vi "Find Non Part Signal Indexes.vi"(0 "All Type Info":T1, 5 "Channels":T3[](array[typedef])) -> (4 "Total Channel Indexes":i32[](array[numeric]), 6 "Non Part Indexes (data)":i32[](array[numeric]), 8 "Non Part Indexes (description)":i32[](array[numeric]))   [LabVIEW 2023]
uses:
  Type Defs and Controls/Channel Config.ctl
  Type Defs and Controls/All Part Info.ctl
  Type Defs and Controls/Part Info.ctl
panel:
  out "Part Channel Indexes":u16[](array[numeric])
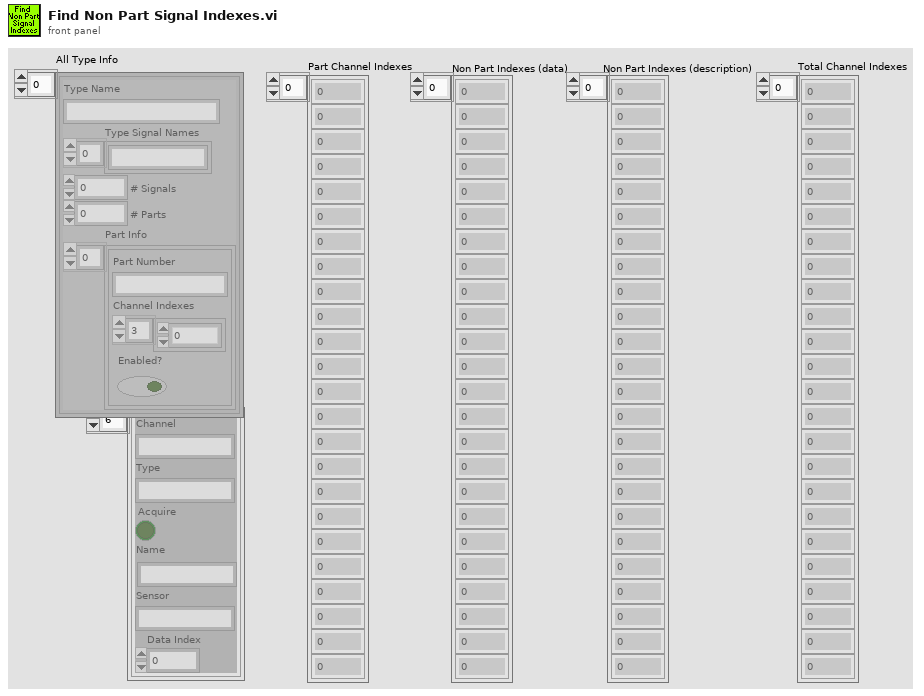
[diagram p1: front panel]
types:
  T1 = typedef "All Part Info.ctl" = cluster{"Type Name":string, "Type Signal Names":string[], "# Signals":i32, "# Parts":i32, "Part Info":T2[]}[]
  T2 = typedef "Part Info.ctl" = cluster{"Part Number":string, "Channel Indexes":u16[], "Enabled?":bool}
  T3 = typedef "Channel Config.ctl" = cluster{"Channel":string, "Type":string, "Acquire":bool, "Name":string, "Sensor":string, "Data Index":u32}
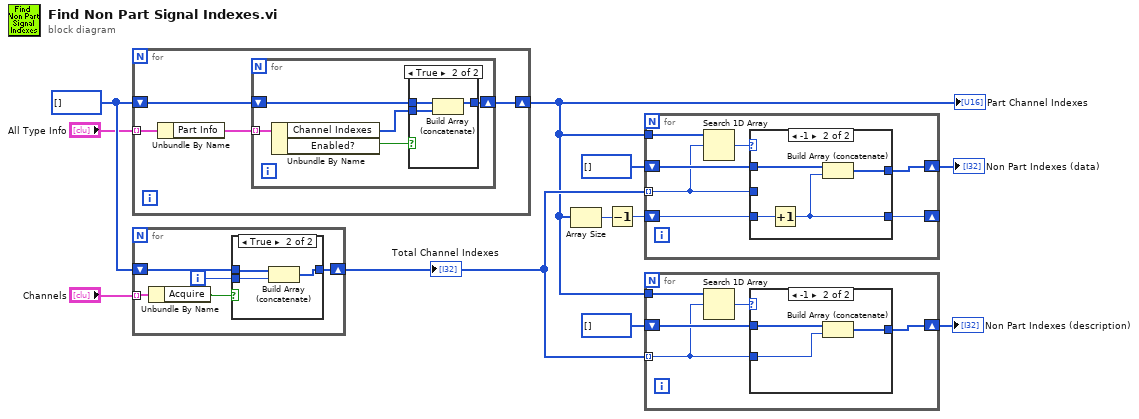
[diagram p0: block diagram]
diagram:
  w8 = u16[] [] ("Channel Indexes")
  n1 = for {
    tunnel: "All Type Info" -> [w15] mode=indexing
    shift-right: [w13] -> w3
    shift-left: w8 -> [w14]
    n2 = Unbundle By Name(w15) -> ("Part Info"=w12:T2[])
    n3 = for {
      tunnel: w12 -> [w20] mode=indexing
      shift-right: [w18] -> w13
      shift-left: w14 -> [w19]
      n4 = Unbundle By Name(w20) -> ("Channel Indexes"=w17:u16[], "Enabled?"=w16:bool)
      n5 = case shown="True" w16 {
        tunnel: w19 -> [w21 w24]
        tunnel: [w21 w23] -> w18
        tunnel: w17 -> [_ w22]
        frame False {
        }
        frame True {
          n6 = Build Array (concatenate)(w24, w22) -> (w23:u16[])
        }
      }
    }
  }
  "Part Channel Indexes" <- w3
  n7 = for {
    tunnel: "Channels" -> [w29] mode=indexing
    shift-right: [w25] -> w4
    shift-left: w8 -> [w27]
    i -> [w26]
    n8 = Unbundle By Name(w29) -> ("Acquire"=w28:bool)
    n9 = case shown="True" w28 {
      tunnel: w27 -> [w30 w33]
      tunnel: w26 -> [_ w32]
      tunnel: [w30 w31] -> w25
      frame False {
      }
      frame True {
        n10 = Build Array (concatenate)(w33, w32) -> (w31:i32[])
      }
    }
  }
  "Total Channel Indexes" <- w4
  n11 = Array Size(array=w3) -> (size(s)=w6:i32)
  n12 = Decrement(x=w6) -> (x-1=w5:i32)
  n13 = for {
    tunnel: w3 -> [w40]
    tunnel: w4 -> [w36] mode=indexing
    shift-right: [w37] -> w10
    shift-left: i32[] [] -> [w38]
    shift-right: [w34] -> _
    shift-left: w5 -> [w35]
    n14 = Search 1D Array(1D array=w40, element=w36) -> (index of element=w39:i32)  [unwired: 1 in]
    n15 = case shown="-1" w39 {
      tunnel: w36 -> [_ _]
      tunnel: w38 -> [w42 w46]
      tunnel: [w42 w45] -> w37
      tunnel: w35 -> [w41 w44]
      tunnel: [w41 w43] -> w34
      frame 0, Default {
      }
      frame -1 {
        n16 = Increment(x=w44) -> (x+1=w43:i32)
        n17 = Build Array (concatenate)(w46, w43) -> (w45:i32[])
      }
    }
  }
  "Non Part Indexes (data)" <- w10
  n18 = for {
    tunnel: w3 -> [w51]
    tunnel: w4 -> [w47] mode=indexing
    shift-right: [w48] -> w2
    shift-left: i32[] [] -> [w49]
    n19 = Search 1D Array(1D array=w51, element=w47) -> (index of element=w50:i32)  [unwired: 1 in]
    n20 = case shown="-1" w50 {
      tunnel: w47 -> [_ w53]
      tunnel: w49 -> [w52 w55]
      tunnel: [w52 w54] -> w48
      frame 0, Default {
      }
      frame -1 {
        n21 = Build Array (concatenate)(w55, w53) -> (w54:i32[])
      }
    }
  }
  "Non Part Indexes (description)" <- w2
